vi "quote String.vi"(8 "Trennzeichen out":string=" ", 9 "Quote":string="\"", 11 "String (Eingang)":string[](array[string])) -> (3 "String (Ausgang)":string)   [LabVIEW 2020, in "Linearisierung v2.lvlib" / "SpanEinstellungen.lvlib"]
uses:
  SpanEinstellungen.lvlib
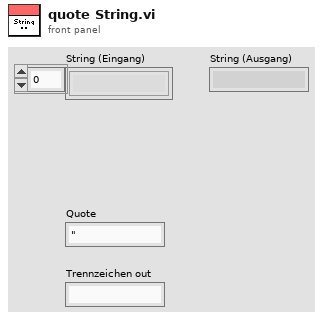
[diagram p1: front panel]
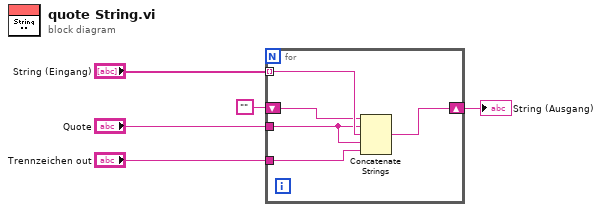
[diagram p0: block diagram]
diagram:
  n1 = for {
    tunnel: "String (Eingang)" -> [w10] mode=indexing
    tunnel: "Quote" -> [w9]
    shift-right: [w8] -> w4
    shift-left: "" -> [w7]
    tunnel: "Trennzeichen out" -> [w6]
    n2 = Concatenate Strings(w7, w9, w10, w9, w6) -> (w8:string)
  }
  "String (Ausgang)" <- w4
